vi "Close.vi"(8 "error in (no error)":errorcluster, 11 "RS232 to GPIB ConvBox in":refnum<class "RS232 to GPIB ConvBox.lvclass">) -> (0 "error out":errorcluster, 3 "RS232 to GPIB ConvBox out":refnum<class "RS232 to GPIB ConvBox.lvclass">)   [LabVIEW 2019, in "Protocols.lvlib" / "RS232 to GPIB ConvBox.lvclass"]
uses:
  RS232 to GPIB ConvBox.lvclass
  RS232 to GPIB ConvBox.lvclass/RS232 to GPIB ConvBox.ctl
  Data Access/Read Port Ref.vi
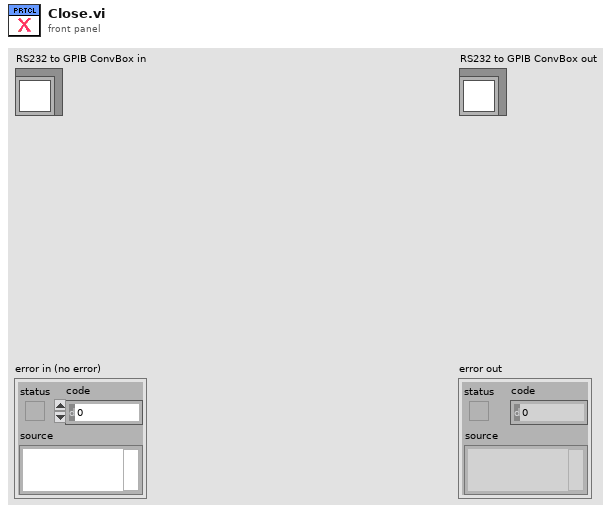
[diagram p1: front panel]
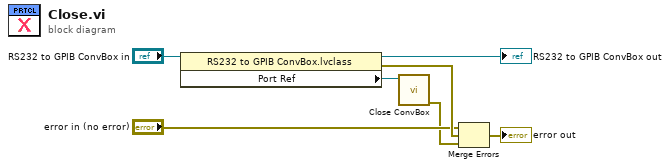
[diagram p0: block diagram]
diagram:
  n1 = property class="RS232 to GPIB ConvBox.lvclass"(reference="RS232 to GPIB ConvBox in") -> (reference out=→"RS232 to GPIB ConvBox out":refnum<class "RS232 to GPIB ConvBox.lvclass">, error out=w7:errorcluster, "Port Ref"=w2:refnum<visa-resource-name>)  [unwired: 1 in]
  n2 = call "Close ConvBox.vi"("Serial Port"=w2) -> ("error out"=w1:errorcluster)  [unwired: 10 in]
  n3 = Merge Errors("error in (no error)", w7, w1) -> (→"error out":errorcluster)
